vi "BreathTrig.vi"(7 "SetUp Mode":bool, 10 "Digitizer Settings":T1={"Digitizer delay (us) "=0.0, "rf points per line"=2048, "lines per plane"=128, "Samp Rate (Hz)"=100000000.0, "Additional dig delay (us)"=0.0, "Voltage Scale"=0.4, "Pre-Looks"=0, "Offset delay (us)"=0.0, "bits A/D"=8, "Avg Num"=1, "DigTimeOut"=5.0, "Rel Dig Delay"=0.0, "Dig Ch"=0, "LeCroyCluster"={"LeCroy Channels"=[TRUE, FALSE, FALSE, FALSE], "LC read pt offset"=0.0, "Sweep Avg"=FALSE}, "Main Digitizer"=enum."NI Digitizer", "Dig Config"=enum."Single channel", "Digitizer ID Cluster"={"Acqiris/Alazar/SP ID"=[], "NI Instr Handles"=[], "LeCroy VISA"="", "GaGe Handle"={"Handle"=0, "Sample size"=0, "Resolution"=0, "Offset"=0, "Channels"=0, "Boards"=0}, "ATS Ref"="ATS9350", "Acqiris Address"=["PCI::INSTR0"], "ADQRef"=refnum, "adq_cu_ptr"=refnum}, "Trigger Settings"={"Trig Source"=1, "Trig Coupling"=0, "Trig Slope"=0, "Level (mV)"=1500.0}, "Bulk Acq"=FALSE, "Bulk Start Indexes"=[], "Data Ref RF"=refnum, "NI ID/Channel"=[], "Total Dig CH"=1, "Xtra Ann Trig delay (us)"=10.0, "Fix Z Delay?"=FALSE, "One Way Transmission?"=FALSE, "Data Ref Log"=refnum} {"Trigger Settings"."Trig Slope" items=["Positive", "Negative"]; "Trigger Settings"."Level (mV)" format="%.2f"; "Trigger Settings"."Trig Coupling" items=["DC 1 MOhm", "AC 1 MOhm", "DC 50 Ohm", "AC 50 Ohm"]; "Trigger Settings"."Trig Source" items=["Chan 1", "External"]; "Rel Dig Delay" format="%.2f"; "DigTimeOut" format="%.2f"; "Avg Num" min=1; "Offset delay (us)" format="%.2f"; "Additional dig delay (us)" format="%.2f"; "Digitizer delay (us)" format="%.2f"}, 11 "Xmit Ring":i16) -> (2 "BINGO":bool)   [LabVIEW 2022 SP3]
uses:
  Digitizers/-DigitizerRoutines/DigitizerSettings.ctl
  Digitizers/-DigitizerRoutines/Digitizer.ctl
  Digitizers/-DigitizerRoutines/DigConfig.ctl
  Digitizers/-DigitizerRoutines/DigitizerID.ctl
  C:/Windows/System32/ADQAPI_dotNet_helper.dll
  Windows/System32/ADQAPI_dotNet_helper.dll
  <vilib>/Platform/TimedLoop/XDataNode/timing_clust.ctl
  <vilib>/Platform/TimedLoop/XDataNode/nitl_modes.ctl
  <vilib>/Platform/TimedLoop/XDataNode/wakeup.ctl
  Motion Controllers/-MotionRoutines/MotionGlobals.vi
  <instrlib>/niScope/Acquire/Fetch/niScope Multi Fetch Binary 8.vi
  <vilib>/Platform/TimedLoop/XDataNode/XDataNode.xnode
  <vilib>/ptbypt/NI_PtbyPt.lvlib
  <instrlib>/Acqiris Dx/Acqiris Dx.lvlib
  <instrlib>/Acqiris Bx/Acqiris Bx.lvlib
  <vilib>/Analysis/NI_AALPro.lvlib
  <vilib>/Analysis/NI_AALBase.lvlib
  <vilib>/Platform/TimedLoop/XDataNode/XDNodeRunTimeDep.lvlib
panel:
  in  "Use Line 6?":bool
  in  "delay (ms)":u32
  out "Trig State":cluster{i16, i32}(graph)
  in  "Exit":bool
  in  "timeout (s)":dbl=1.0 format="%.2f"
  in  "neg cross":dbl=-3.0
  in  "Time between RF trace (ms)":u32=5
  in  "initial Skip index":i32=50
  in  "Zero Crossing":enum16{"either", "minus-plus", "plus-minus"}(ring)=enum."minus-plus"
  in  "AS Med Fil":i32=20
  out "Waveform Graph":dbl[](graph)
  out "Smooth Chart":dbl(graph)
  in  "RF Thresh":i32=15
  in  "ThreshMed Lgth":i32=8
  in  "RF PTs":i32=1000
  out "Raw and smoothed data":dbl[](graph)
  # "Pts to acquire for Breath RF trace"
  # "Skip intial points in RF trace"
  # "software based PRF"
  # "right rank for Envelope med filter"
  # "Simple threshold to find chest"
  # "White is zero crossing and red is delayed trigger"
  # "Length of pt-pt median filter"
  # "Zero Crossing"
  # "minumum crossing before valid trigger"
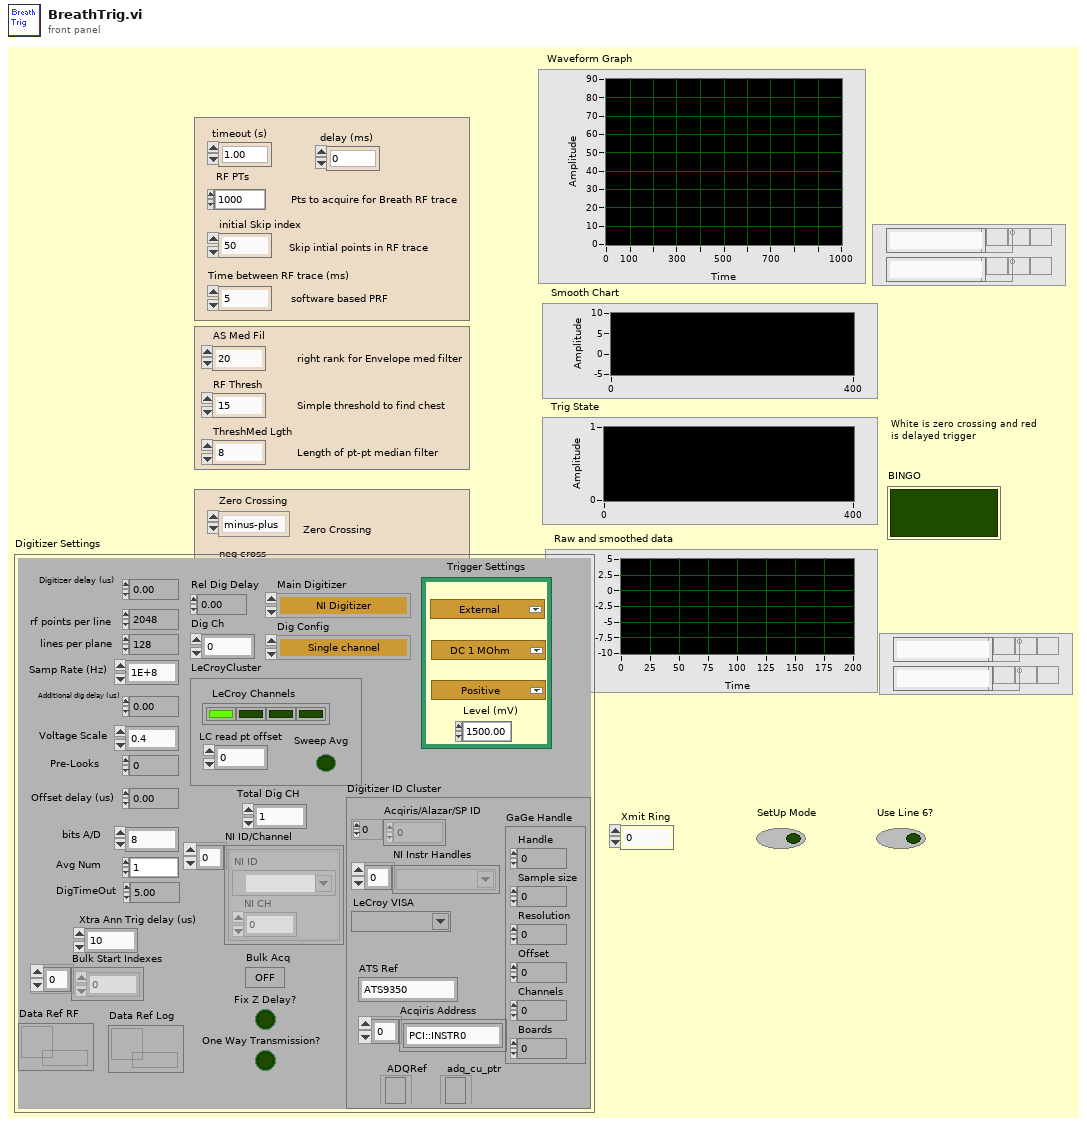
[diagram p1: front panel]
types:
  T1 = typedef "DigitizerSettings.ctl" = cluster{"Digitizer delay (us) ":dbl, "rf points per line":i32, "lines per plane":i32, "Samp Rate (Hz)":dbl, "Additional dig delay (us)":dbl, "Voltage Scale":dbl, "Pre-Looks":i32, "Offset delay (us)":dbl, "bits A/D":i8, "Avg Num":i32, "DigTimeOut":sgl, "Rel Dig Delay":sgl, "Dig Ch":i32, "LeCroyCluster":cluster{"LeCroy Channels":bool[], "LC read pt offset":dbl, "Sweep Avg":bool}, "Main Digitizer":T2, "Dig Config":T3, "Digitizer ID Cluster":T4, "Trigger Settings":cluster{"Trig Source":u16, "Trig Coupling":u16, "Trig Slope":u16, "Level (mV)":dbl}, "Bulk Acq":bool, "Bulk Start Indexes":i32[], "Data Ref RF":refnum<data-value>, "NI ID/Channel":cluster{"NI ID":refnum<k15>, "NI CH":i32}[], "Total Dig CH":i32, "Xtra Ann Trig delay (us)":dbl, "Fix Z Delay?":bool, "One Way Transmission?":bool, "Data Ref Log":refnum<data-value>}
  T2 = typedef "Digitizer.ctl" = enum16{"Acqiris Digitizer", "NI Digitizer", "LeCroy", "GaGe", "AlazarTech", "No Digitizer", "Teledyne"}
  T3 = typedef "DigConfig.ctl" = enum16{"Single channel", "2 Chans w/ 2 Acqiris", "2 Chans w/ 1 Acqiris", "5-CH Pulser New", "5-CH pulser w/ ann array", "5-pass style ann array", "Empty"}
  T4 = typedef "DigitizerID.ctl" = cluster{"Acqiris/Alazar/SP ID":u32[], "NI Instr Handles":refnum<k15>[], "LeCroy VISA":refnum<visa-resource-name>, "GaGe Handle":cluster{"Handle":u32, "Sample size":u32, "Resolution":i32, "Offset":i32, "Channels":u32, "Boards":u32}, "ATS Ref":string, "Acqiris Address":string[], "ADQRef":refnum<k24>, "adq_cu_ptr":refnum<k24>}
  T5 = typedef "Breath_Mode.ctl" = u16
  T6 = typedef "EKG_Mode.ctl" = u16
  T7 = typedef "XDNodeRunTimeDep.lvlib/timing_clust.ctl" = cluster{"Expected End [f-1]":u64, "Actual End [f-1]":u64, "Finished Late? [f-1]":bool, "Expected End [i-1]":u64, "Actual End [i-1]":u64, "Finished Late? [i-1]":bool, "Expected Start [i]":u64, "Actual Start [i]":u64, "Expected Start [f]":u64, "Actual Start [f]":u64, "Source Name":string, "Structure Name":string, "Period":i64, "Deadline":i64, "Offset":i64, "Start":i64, "Priority":i32, "Timeout":i32, "Mode":T8, "Wakeup Reason":T9, "Error":errorcluster, "Source Type":string, "Secondary Source Type":string, "Global End Time":u64, "Global Start Time":u64, "Frame Duration":u64, "Iteration Duration":u64, "Assigned CPU":i32, "I/O Scan Engine Mode":u32}
  T8 = typedef "XDNodeRunTimeDep.lvlib/nitl_modes.ctl" = enum32{"No Change", "Process missed periods, maintain original phase", "Discard missed periods, maintain original phase", "Process missed periods, ignore original phase", "Discard missed periods, ignore original phase"}
  T9 = typedef "XDNodeRunTimeDep.lvlib/wakeup.ctl" = enum32{"Normal", "Aborted", "Asynchronous wakeup", "Timing source error", "Timed loop error", "Timeout"}
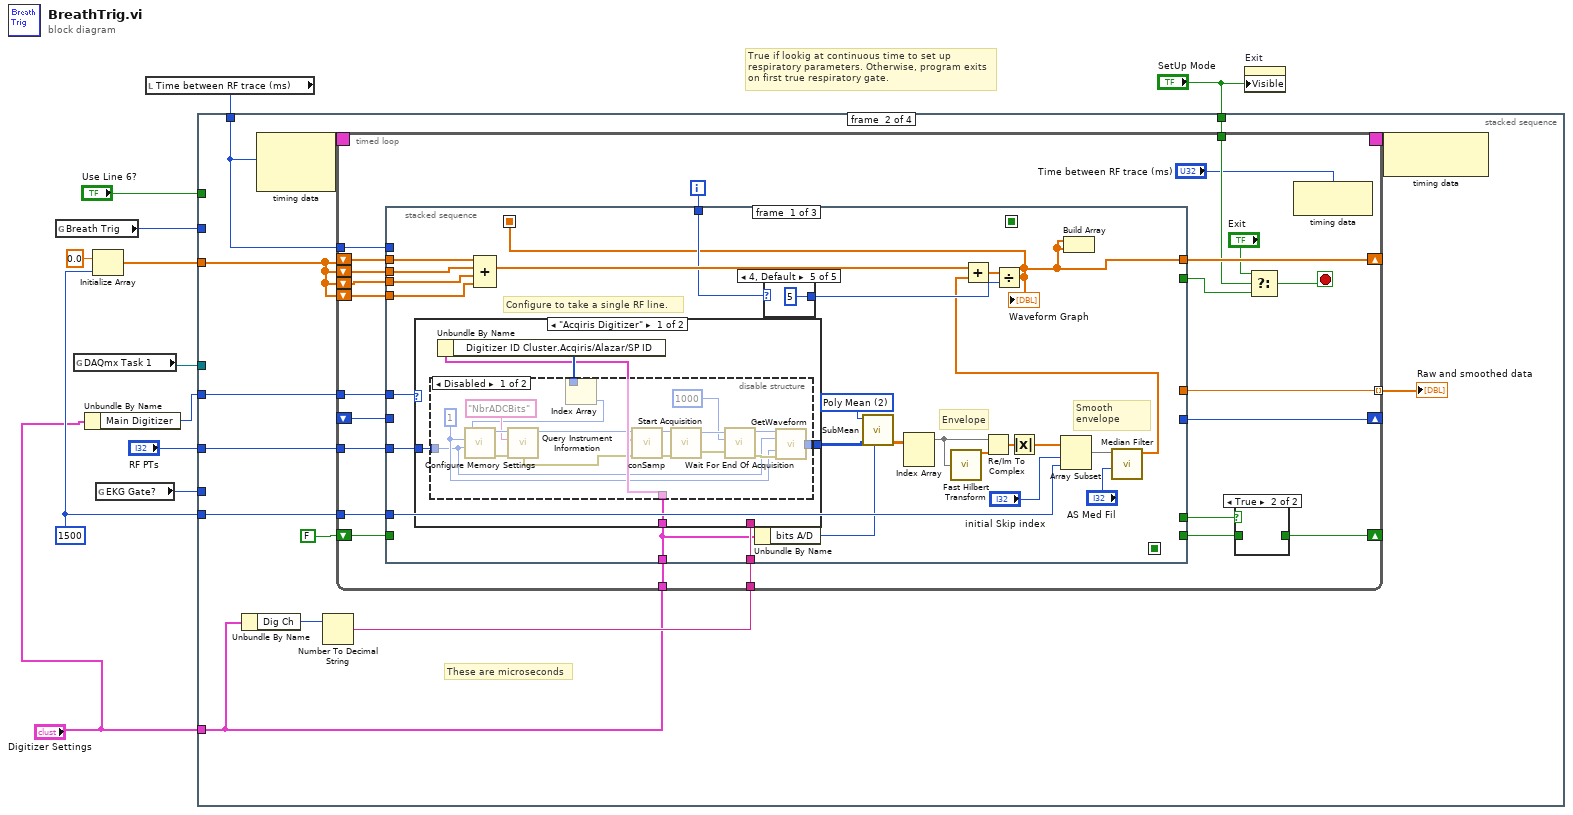
[diagram p0: block diagram]
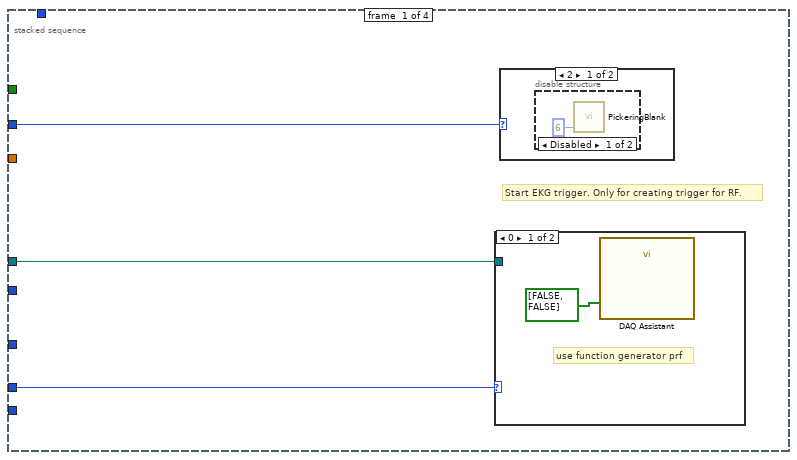
[diagram p2: hidden frame]
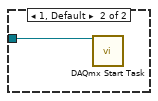
[diagram p5: hidden frame]
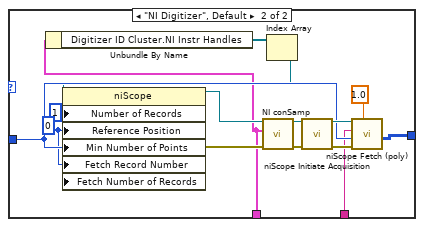
[diagram p8: hidden frame]
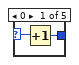
[diagram p9: hidden frame]
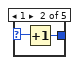
[diagram p10: hidden frame]
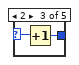
[diagram p11: hidden frame]
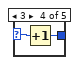
[diagram p12: hidden frame]
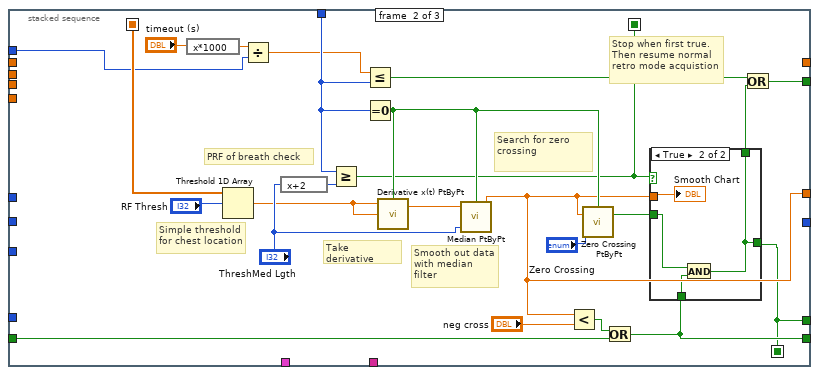
[diagram p13: hidden frame]
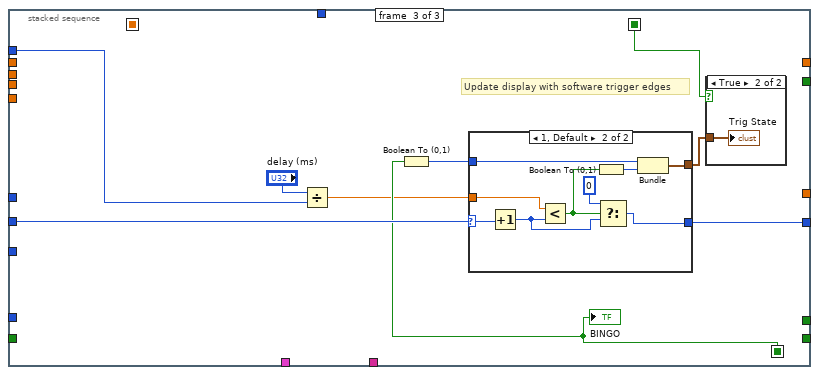
[diagram p15: hidden frame]
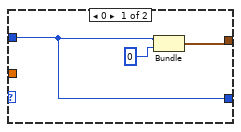
[diagram p17: hidden frame]
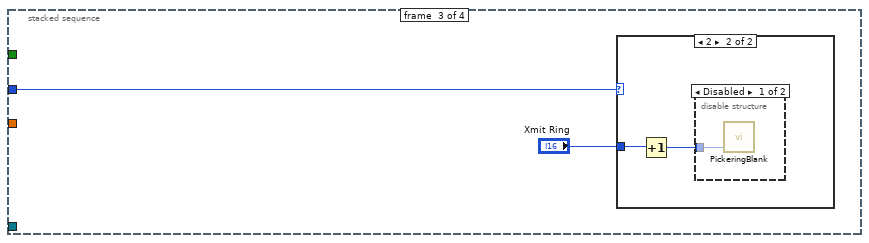
[diagram p18: hidden frame]
diagram:
  w9 = 1500
  # "True if lookig at continuous time to set up respiratory parameters. Otherwise, program exits on first true respiratory gate."
  n1 = global read "MotionGlobals.vi" "Breath Trig"() -> (w7:T5)
  n2 = global read "MotionGlobals.vi" "DAQmx Task 1"() -> (w6:refnum<k21>)
  n3 = Unbundle By Name("Digitizer Settings") -> ("Main Digitizer"=w1:T2)
  n4 = Initialize Array(0.0 ("element"), w9) -> (w12:dbl[])
  n5 = global read "MotionGlobals.vi" "EKG Gate?"() -> (w3:T6)
  n6 = local read "Time between RF trace (ms)"() -> (w4:u32)
  n7 = stacked-sequence {
    tunnel: w6 -> [w15 _ _ w194]
    tunnel: "RF PTs" -> [_ w31 _ _]
    tunnel: w12 -> [_ w28 _ _]
    tunnel: w9 -> [_ w29 _ _]
    tunnel: w1 -> [_ w26 _ _]
    tunnel: "SetUp Mode" -> [_ w24 _ w193]
    tunnel: w7 -> [w14 _ w187 _]
    tunnel: "Use Line 6?" -> [_ _ _ _]
    tunnel: w4 -> [_ w21 _ _]
    tunnel: w3 -> [w13 _ _ w192]
    tunnel: "Digitizer Settings" -> [_ w20 _ _]
    frame #0 {
      # "Start EKG trigger. Only for creating trigger for RF."
      n8 = case shown="0" w13 {
        tunnel: w15 -> [_ w18]
        frame 0 {
          # "use function generator prf"
          n9 = call "DAQ Assistant"("data"=bool[] [FALSE, FALSE]) -> ()  [unwired: 3 in, 16 out]
        }
        frame 1, Default {
          n10 = call <vilib>:"DAQmx Start Task.vi"("task/channels in"=w18) -> ()  [unwired: 1 in, 14 out]
        }
      }
      n11 = case shown="2" w14 {
        frame 2 {
          n12 = disable-structure shown="Disabled" {
            frame Disabled {
              n13 = call "PickeringBlank.vi"("Xmit Ring"=i8 6) -> ()  [unwired: 5 out]
            }
            frame Enabled {
            }
          }
        }
        frame 0, Default {
        }
      }
    }
    frame #1 {
      # "These are microseconds"
      n14 = Unbundle By Name(w20) -> ("Dig Ch"=w19:i32)
      n15 = node-c288(w21) -> (w23:T7)  [unwired: 1 out]
      n16 = Number To Decimal String(number=w19) -> (decimal integer string=w25:string)  [unwired: 1 out]
      n17 = timed-loop {
        tunnel: [w53] -> w30 mode=indexing
        tunnel: w31 -> [w55]
        shift-right: [w49] -> _
        shift-left: w28 -> [w52]
        shift-left: w28 -> [w51]
        shift-left: w28 -> [w50]
        tunnel: w29 -> [w48]
        shift-left: w28 -> [w47]
        shift-right: [w37] -> _
        shift-left: FALSE -> [w46]
        tunnel: w26 -> [w45]
        tunnel: w25 -> [w44]
        tunnel: w24 -> [w43]
        shift-right: [w39] -> _
        shift-left: _ -> [w40]
        timing: w23 -> [_]
        timing-out: [_] -> w22
        tunnel: w21 -> [w34]
        tunnel: w20 -> [w32]
        i -> [w54]
        stop <- w42 stop-if-true
        n18 = stacked-sequence {
          seq-local: [w62 _ _] -> [_ w154 _]
          seq-local: [_ w133 _] -> [_ _ w166]
          seq-local: [_ w134 _] -> [_ _ w161]
          tunnel: w55 -> [w83 _ _]
          tunnel: w54 -> [w73 w147 _]
          tunnel: [_ w140 _] -> w53
          tunnel: w52 -> [w78 _ _]
          tunnel: w51 -> [w77 _ _]
          tunnel: w50 -> [w76 _ _]
          tunnel: [w62 _ _] -> w49
          tunnel: [_ w151 _] -> w38
          tunnel: w48 -> [w68 _ _]
          tunnel: w47 -> [w67 _ _]
          tunnel: w46 -> [_ w141 _]
          tunnel: [_ w138 _] -> w36
          tunnel: w45 -> [w66 _ _]
          tunnel: w44 -> [w64 _ _]
          tunnel: [_ _ w165] -> w39
          tunnel: w40 -> [_ _ w168]
          tunnel: [_ w133 _] -> w35
          tunnel: w34 -> [_ w132 w160]
          tunnel: w32 -> [w61 _ _]
          frame #0 {
            w85 = u16 2 items=["Mean from lines", "Mean just lines", "Poly Mean", "No mean"] ("Type of Mean")
            # "Smooth envelope"
            # "Envelope"
            # "Configure to take a single RF line."
            n19 = case shown="\"Acqiris Digitizer\"" w66 {
              tunnel: w83 -> [w89 w116]
              tunnel: [w88 w111] -> w82
              tunnel: w64 -> [_ w112]
              tunnel: w61 -> [w86 w108]
              frame "Acqiris Digitizer" {
                n20 = Unbundle By Name(w86) -> ("Digitizer ID Cluster.Acqiris/Alazar/SP ID"=w87:u32[])
                n21 = disable-structure shown="Disabled" {
                  disable-tunnel: w89 -> [w97 _]
                  disable-tunnel: [w96 _] -> w88
                  disable-tunnel: w87 -> [w92 _]
                  disable-tunnel: w86 -> [w90 _]
                  frame Disabled {
                    w98 = 1 ("Number of Segments (1)")
                    n22 = Index Array(array=w92) -> (element=w91:u32)  [unwired: 1 in]
                    n23 = call <instrlib>:"Configure Memory Settings.vi"("Number of Samples (1000)"=w97, "Number of Segments (1)"=w98, "Instrument ID"=w91) -> ("error out"=w106:errorcluster, "dup Instrument ID"=w104:u32)  [unwired: 1 in, 2 out]
                    n24 = call <instrlib>:"Query Instrument Information.vi"("Instrument ID"=w104, "Parameter String"="NbrADCBits", "error in (no error)"=w106) -> ("dup Instrument ID"=w94:u32, "error out"=w93:errorcluster)  [unwired: 1 in, 4 out]
                    n25 = call "conSamp.vi"("error in"=w93, "Digitizer Settings"=w90, "InstrumentID"=w94) -> ("error out"=w105:errorcluster, "DUP ID"=w107:u32)  [unwired: 1 in]
                    n26 = call <instrlib>:"Start Acquisition.vi"("error in (no error)"=w105, "Instrument ID"=w107) -> ("error out"=w101:errorcluster, "dup Instrument ID"=w102:u32)  [unwired: 2 in]
                    n27 = call <instrlib>:"Wait For End Of Acquisition.vi"("error in (no error)"=w101, "Timeout"=1000, "Instrument ID"=w102) -> ("error out"=w99:errorcluster, "dup Instrument ID"=w100:u32)  [unwired: 3 out]
                    n28 = call "GetWaveform.vi"("Acq ID Out"=w100, "Num Samps"=w97, "Num Segs"=w98, "error in"=w99) -> ("Acquired Waveform16 bit"=w96:i16[][])  [unwired: 2 in, 9 out]
                  }
                  frame Enabled {
                  }
                }
              }
              frame "NI Digitizer", Default {
                w114 = 1
                w115 = 0
                n29 = Unbundle By Name(w108) -> ("Digitizer ID Cluster.NI Instr Handles"=w109:refnum<k15>[])
                n30 = Index Array(array=w109) -> (element=w110:refnum<k15>)  [unwired: 1 in]
                n31 = property class="niScope"(reference=w110, "Number of Records"=w114, "Reference Position"=w115, "Min Number of Points"=w116, "Fetch Record Number"=w115, "Fetch Number of Records"=w114) -> (reference out=w120:refnum<k15>, error out=w119:errorcluster)  [unwired: 1 in]
                n32 = call "NI conSamp.vi"("error in"=w119, "Digitizer Settings"=w108, "InstrumentID"=w120) -> ("error out"=w122:errorcluster, "DUP ID"=w121:refnum<k15>)  [unwired: 1 in]
                n33 = call <instrlib>:"niScope Initiate Acquisition.vi"("instrument handle"=w121, "error in"=w122) -> ("instrument handle out"=w118:refnum<k15>, "error out"=w117:errorcluster)  [unwired: 1 in, 11 out]
                n34 = call-poly <instrlib>:"niScope Fetch (poly).vi"("timeout"=1.0, "error in"=w117, "numSamples"=w116, "channels"=w112, "instrument handle"=w118) -> ("wfm"=w111:i8[][])  [unwired: 6 out]
              }
            }
            n35 = Compound Arithmetic op=ADD(w78, w77, w76, w67) -> (w75:dbl[])
            n36 = Unbundle By Name(w61) -> ("bits A/D"=w60:i8)
            n37 = case shown="4, Default" w73 {
              selector: w73 -> [w124 w126 w128 w130 _]
              tunnel: [w123 w125 w127 w129 5] -> w72
              frame 0 {
                n38 = Increment(x=w124) -> (x+1=w123:i32)
              }
              frame 1 {
                n39 = Increment(x=w126) -> (x+1=w125:i32)
              }
              frame 2 {
                n40 = Increment(x=w128) -> (x+1=w127:i32)
              }
              frame 3 {
                n41 = Increment(x=w130) -> (x+1=w129:i32)
              }
              frame 4, Default {
              }
            }
            n42 = call "SubMean.vi"("Bit Depth"=w60, "Scan Data In"=w82, "Type of Mean"=w85) -> ("Array"=w84:dbl[][])  [unwired: 3 in, 2 out]
            n43 = Index Array(array=w84) -> (element=w79:dbl[])  [unwired: 2 in]
            n44 = call <vilib>:"Fast Hilbert Transform.vi"("X"=w79) -> ("Hilbert{X}"=w80:dbl[])  [unwired: 1 out]
            n45 = Re/Im To Complex(1:w80, 2:w79) -> (0:w81:cdb[])
            n46 = Absolute Value(x=w81) -> (abs(x)=w71:dbl[])
            n47 = Array Subset(array=w71, index="initial Skip index", length=w68) -> (w70:dbl[])
            n48 = call <vilib>:"Median Filter.vi"("right rank"="AS Med Fil", "X"=w70) -> ("Filtered X"=w69:dbl[])  [unwired: 1 in, 8 out]
            n49 = Add(x=w75, y=w69) -> (x+y=w74:dbl[])
            n50 = Divide(x=w74, y=w72) -> (x/y=w62:dbl[])
            "Waveform Graph" <- w62
            n51 = Build Array(w62, w62) -> ()  [unwired: 1 out]
          }
          frame #1 {
            # "PRF of breath check"
            # "Search for zero crossing"
            # "Smooth out data with median filter"
            # "Take derivative"
            # "Stop when first true. Then resume normal retro mode acquistion"
            # "Simple threshold for chest location"
            n52 = expression code="x*1000"("timeout (s)") -> (w136:dbl)
            n53 = Threshold 1D Array(2:"RF Thresh", 3:w154) -> (0:w146:dbl)  [unwired: 1 out]
            n54 = Divide(x=w136, y=w132) -> (x/y=w135:dbl)
            n55 = expression code="x+2"("ThreshMed Lgth") -> (w149:i32)
            n56 = Greater Or Equal?(x=w147, y=w149) -> (x >= y?=w134:bool)
            n57 = Less Or Equal?(x=w135, y=w147) -> (x <= y?=w153:bool)
            n58 = Equal To 0?(x=w147) -> (x = 0?=w143:bool)
            n59 = call <vilib>:"Derivative x(t) PtByPt.vi"("initialize"=w143, "initial condition"=w146, "x"=w146) -> ("dx/dt"=w148:dbl)  [unwired: 1 in, 1 out]
            n60 = call <vilib>:"Median PtByPt.vi"("initialize"=w143, "sample length"="ThreshMed Lgth", "x"=w148) -> ("median"=w140:dbl)  [unwired: 2 out]
            n61 = Less?(x=w140, y="neg cross") -> (x < y?=w139:bool)
            n62 = call <vilib>:"Zero Crossing PtByPt.vi"("initialize"=w143, "direction"="Zero Crossing", "input data point"=w140) -> ("crossing"=w145:bool)
            n63 = Or(x=w139, y=w141) -> (x .or. y?=w138:bool)
            n64 = case shown="True" w134 {
              tunnel: [_ w156] -> w152
              tunnel: w140 -> [_ w159]
              tunnel: w145 -> [_ w158]
              tunnel: w138 -> [_ w157]
              tunnel: [_ w156] -> w133
              frame False {
              }
              frame True {
                n65 = And(x=w158, y=w157) -> (x .and. y?=w156:bool)
                "Smooth Chart" <- w159
              }
            }
            n66 = Or(x=w153, y=w152) -> (x .or. y?=w151:bool)
          }
          frame #2 {
            # "Update display with software trigger edges"
            n67 = Divide(x="delay (ms)", y=w160) -> (x/y=w164:dbl)
            n68 = Boolean To (0,1)(Boolean=w166) -> (0, 1=w163:i16)
            n69 = case shown="1, Default" w168 {
              selector: w168 -> [_ w181]
              tunnel: [w171 w179] -> w165
              tunnel: w164 -> [_ w180]
              tunnel: w163 -> [w171 w174]
              tunnel: [w170 w175] -> w162
              frame 0 {
                n70 = Bundle(w171, 0) -> (w170:cluster{i16, i32})  [unwired: 1 out]
              }
              frame 1, Default {
                n71 = Increment(x=w181) -> (x+1=w178:i32)
                n72 = Less?(x=w180, y=w178) -> (x < y?=w176:bool)
                n73 = Boolean To (0,1)(Boolean=w176) -> (0, 1=w173:i16)
                n74 = Select(t=0, s=w176, f=w178) -> (s? t:f=w179:i32)
                n75 = Bundle(w174, w173) -> (w175:cluster{i16, i16})  [unwired: 1 out]
              }
            }
            n76 = case shown="True" w161 {
              tunnel: w162 -> [_ w169]
              frame False {
              }
              frame True {
                "Trig State" <- w169
              }
            }
            "BINGO" <- w166
          }
        }
        n77 = case shown="True" w35 {
          tunnel: [w59 _] -> w37
          tunnel: w36 -> [w59 _]
          frame False {
          }
          frame True {
          }
        }
        n78 = Select(t="Exit", s=w43, f=w38) -> (s? t:f=w42:bool)
        n79 = node-c288("Time between RF trace (ms)") -> ()  [unwired: 1 out]
      }
      "Raw and smoothed data" <- w30
      n80 = node-c288(w22) -> ()  [unwired: 1 out]
    }
    frame #2 {
      n81 = case shown="2" w187 {
        tunnel: "Xmit Ring" -> [_ w190]
        frame 0, Default {
        }
        frame 2 {
          n82 = Increment(x=w190) -> (x+1=w189:i16)
          n83 = disable-structure shown="Disabled" {
            disable-tunnel: w189 -> [w191 _]
            frame Disabled {
              n84 = call "PickeringBlank.vi"("Xmit Ring"=w191) -> ()  [unwired: 5 out]
            }
            frame Enabled {
            }
          }
        }
      }
    }
    frame #3 {
      n85 = case shown="False" w193 {
        tunnel: w194 -> [w197 _]
        tunnel: w192 -> [w195 _]
        frame False {
          # "Add in selected delay after zero crossing"
          n86 = local read "delay (ms)"() -> (w196:u32)
          n87 = case shown="0" w195 {
            tunnel: w197 -> [_ w200]
            frame 0 {
              # "turn off function generator prf"
              n88 = call "DAQ Assistant2"("data"=bool[] [TRUE, FALSE]) -> ()  [unwired: 3 in, 16 out]
            }
            frame 1, Default {
              n89 = call <vilib>:"DAQmx Stop Task.vi"("task/channels in"=w200) -> ()  [unwired: 1 in, 14 out]
            }
          }
          n90 = case shown="1, Default" w196 {
            selector: w196 -> [_ w198]
            frame 0 {
            }
            frame 1, Default {
              n91 = Wait (ms)(milliseconds to wait=w198) -> ()  [unwired: 1 out]
            }
          }
        }
        frame True {
        }
      }
    }
  }
  n92 = property on="Exit" class="Bool"("Visible"="SetUp Mode") -> ()  [unwired: 2 in, 2 out]
